vi "Aim_At_Target.vi"() -> ()   [LabVIEW 2019]
uses:
  <vilib>/Rock Robotics/WPI/Joystick/XBox Buttons Indexer.ctl
  <vilib>/Rock Robotics/WPI/Joystick/XBox Axes Indexer.ctl
  <vilib>/Rock Robotics/WPI/ThirdParty/JAS_Junk/TrajLib/PIDController_AtSetpoint.vi
  <vilib>/Rock Robotics/WPI/ThirdParty/JAS_Junk/TrajLib/PIDController_SetPIDF.vi
  <vilib>/Rock Robotics/WPI/ThirdParty/JAS_Junk/TrajLib/PIDController_SetDerivativeFilter.vi
  <vilib>/Rock Robotics/WPI/ThirdParty/JAS_Junk/TrajLib/PIDController_SetIntegratorRange.vi
  <vilib>/Rock Robotics/WPI/ThirdParty/JAS_Junk/TrajLib/PIDController_SetTolerancePandV.vi
  <vilib>/Rock Robotics/WPI/ThirdParty/JAS_Junk/TrajLib/PIDController_DisableContinousInput.vi
  <vilib>/Rock Robotics/WPI/ThirdParty/JAS_Junk/TrajLib/PIDController_EnableContinousInput.vi
  <vilib>/Rock Robotics/WPI/ThirdParty/JAS_Junk/TrajLib/PIDController_Reset.vi
  <vilib>/Rock Robotics/WPI/ThirdParty/JAS_Junk/TrajLib/PIDController_New.vi
  <vilib>/Rock Robotics/WPI/ThirdParty/JAS_Junk/TrajLib/PIDController_SetOutputLimits.vi
  <vilib>/Rock Robotics/WPI/ThirdParty/JAS_Junk/TrajLib/PIDController_NewPeriod.vi
  <vilib>/Rock Robotics/SystemInterfaces/NetworkCommunication/NetComm_UsageReport_report.vi
  <vilib>/Rock Robotics/WPI/Utilities/WPI_GetSetVariantRefNum.vi
  <vilib>/Rock Robotics/Network Tables/NT Write Boolean.vi
  <vilib>/Rock Robotics/WPI/Joystick/WPI_JoystickArcadeMapping.vi
  <vilib>/Rock Robotics/Network Tables/NT Write Number.vi
  <vilib>/Rock Robotics/WPI/ThirdParty/JAS_Junk/TrajLib/Util_LibraryGlobals.vi
  <vilib>/Rock Robotics/WPI/ThirdParty/JAS_Junk/TrajLib/PIDController_AdvCalculate_FF_Sp_Pv.vi
  <vilib>/Rock Robotics/Network Tables/NT Write Numeric Array.vi
  <vilib>/Rock Robotics/WPI/ThirdParty/PhotonVisionLib/PhotonVisionLib.lvlib
  <vilib>/Rock Robotics/WPI/ThirdParty/JAS_Junk/TrajLib/Trajectory_Library.lvlib
panel:
  in  "Fiiducial ID":i32
  in  "Use Fiducial\nID":bool
  out "Auto Aim\nSelected":bool
  out "TargetFound":bool
  out "Yaw":dbl
  out "DistanceToTarget Meters":dbl
  out "Right Motor Demand":dbl format="%14.4f"
  out "Left Motor Demand":dbl format="%14.4f"
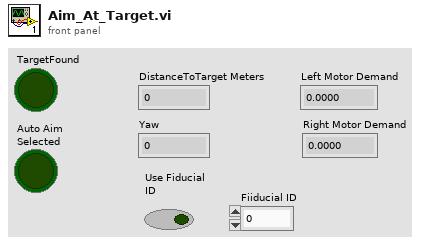
[diagram p1: front panel]
types:
  T1 = typedef "WPI_RobotDriveDevRef.ctl" = cluster{"DevStatus":errorcluster, "Motors[]":T2[], "Square Inputs":bool, "Max Output":dbl}
  T2 = typedef "WPI_MotorControlDeviceRef.ctl" = cluster{"DeviceStatus":errorcluster, "Type":T3, "PWM":cluster{"PWM Channel":T4, "DeadBand":T5}, "CAN":cluster{"Device Number":u8, "SetOutput VI Ref":variant, "GetOutput VI Ref":variant, "Enable VI Ref":variant, "Disable VI Ref":variant, "Data":variant}, "Invert":bool, "DIO PWM":cluster{"PWM \"Enable\" Channel":T4, "DIOChannel":T6, "PWM Rate":dbl}}
  T3 = typedef "WPI_MotorControlType.ctl" = enum16{"PWM", "CAN", "DIO PWM"}
  T4 = typedef "FPGA_DIOPWMChannel.ctl" = enum8{"PWM 0", "PWM 1", "PWM 2", "PWM 3", "PWM 4", "PWM 5", "PWM 6", "PWM 7", "PWM 8", "PWM 9", "PWM MXP 0", "PWM MXP 1", "PWM MXP 2", "PWM MXP 3", "PWM MXP 4", "PWM MXP 5", "PWM MXP 6", "PWM MXP 7", "PWM MXP 8", "PWM MXP 9", "Invalid"}
  T5 = typedef "WPI_PWMDeadband.ctl" = cluster{"Name":string, "maxPositivePwm":i32, "minPositivePwm":i32, "centerPwm":i32, "maxNegativePwm":i32, "minNegativePwm":i32, "angularRange":u16}
  T6 = typedef "FPGA_DIOChannel.ctl" = enum8{"DIO 0", "DIO 1", "DIO 2", "DIO 3", "DIO 4", "DIO 5", "DIO 6", "DIO 7", "DIO 8", "DIO 9", "DIO MXP 0", "DIO MXP 1", "DIO MXP 2", "DIO MXP 3", "DIO MXP 4", "DIO MXP 5", "DIO MXP 6", "DIO MXP 7", "DIO MXP 8", "DIO MXP 9", "DIO MXP 10", "DIO MXP 11", "DIO MXP 12", "DIO MXP 13", "DIO MXP 14", "DIO MXP 15", "SPI Port CS1", "SPI Port CS2", "SPI Port CS3", "SPI Port MISO", "SPI Port MOSI", "Invalid"}
  T7 = typedef "WPI_JoystickDevRef.ctl" = cluster{"Device":T8}
  T8 = typedef "WPI_JoystickDeviceEnum.ctl" = enum16{"USB 0", "USB 1", "USB 2", "USB 3", "USB 4", "USB 5"}
  T9 = typedef "XBox Axes Indexer.ctl" = enum16{"Left X", "Left Y", "Left Trigger", "Right Trigger", "Right X", "Right Y"}
  T10 = typedef "XBox Buttons Indexer.ctl" = enum16{"A", "B", "X", "Y", "Left Bumper", "Right Bumper", "Back", "Start", "Left Joystick", "Right Joystick"}
  T11 = typedef "PhotonVisionLib.lvlib/PhotonPipelineResultType.ctl" = cluster{"TargetCount":i32, "Latency_MilliSec":dbl, "Targets":T12[], "TimeStampSec":dbl}
  T12 = typedef "PhotonVisionLib.lvlib/PhotonTrackedTargetType.ctl" = cluster{"Yaw":dbl, "Pitch":dbl, "Area":dbl, "Skew":dbl, "MinAreaRectCorners":T13[], "BestCameraToTarget":T14, "FiiducialId":i32, "AltCameraToTarget":T14, "PoseAmbiguity":dbl, "DetectedCorners":T13[]}
  T13 = typedef "PhotonVisionLib.lvlib/TargetCornerType.ctl" = cluster{"X":dbl, "Y":dbl}
  T14 = typedef "Trajectory_Library.lvlib/TRANSFORM3D.ctl" = cluster{"TRANSLATION3D":T15, "ROTATION3D":T16, "XF":bool}
  T15 = typedef "Trajectory_Library.lvlib/TRANSLATION3D.ctl" = cluster{"X":dbl, "Y":dbl, "Z":dbl}
  T16 = typedef "Trajectory_Library.lvlib/ROTATION3D.ctl" = cluster{"Q_quaternion":T17}
  T17 = typedef "Trajectory_Library.lvlib/QUATERNION.ctl" = cluster{"R":dbl, "V":dbl[]}
  T18 = typedef "Trajectory_Library.lvlib/PID_ADV_LIMITS.ctl" = cluster{"MaxInput":dbl, "MinInput":dbl, "Continuous":bool, "MaxOutput":dbl, "MinOutput":dbl}
  T19 = typedef "Trajectory_Library.lvlib/PID_ADV_TUNING.ctl" = cluster{"Kf":dbl, "Kp":dbl, "Ki":dbl, "Kd":dbl, "MaximumIntegral":dbl, "MinimumIntegral":dbl, "Filter Derivative":bool}
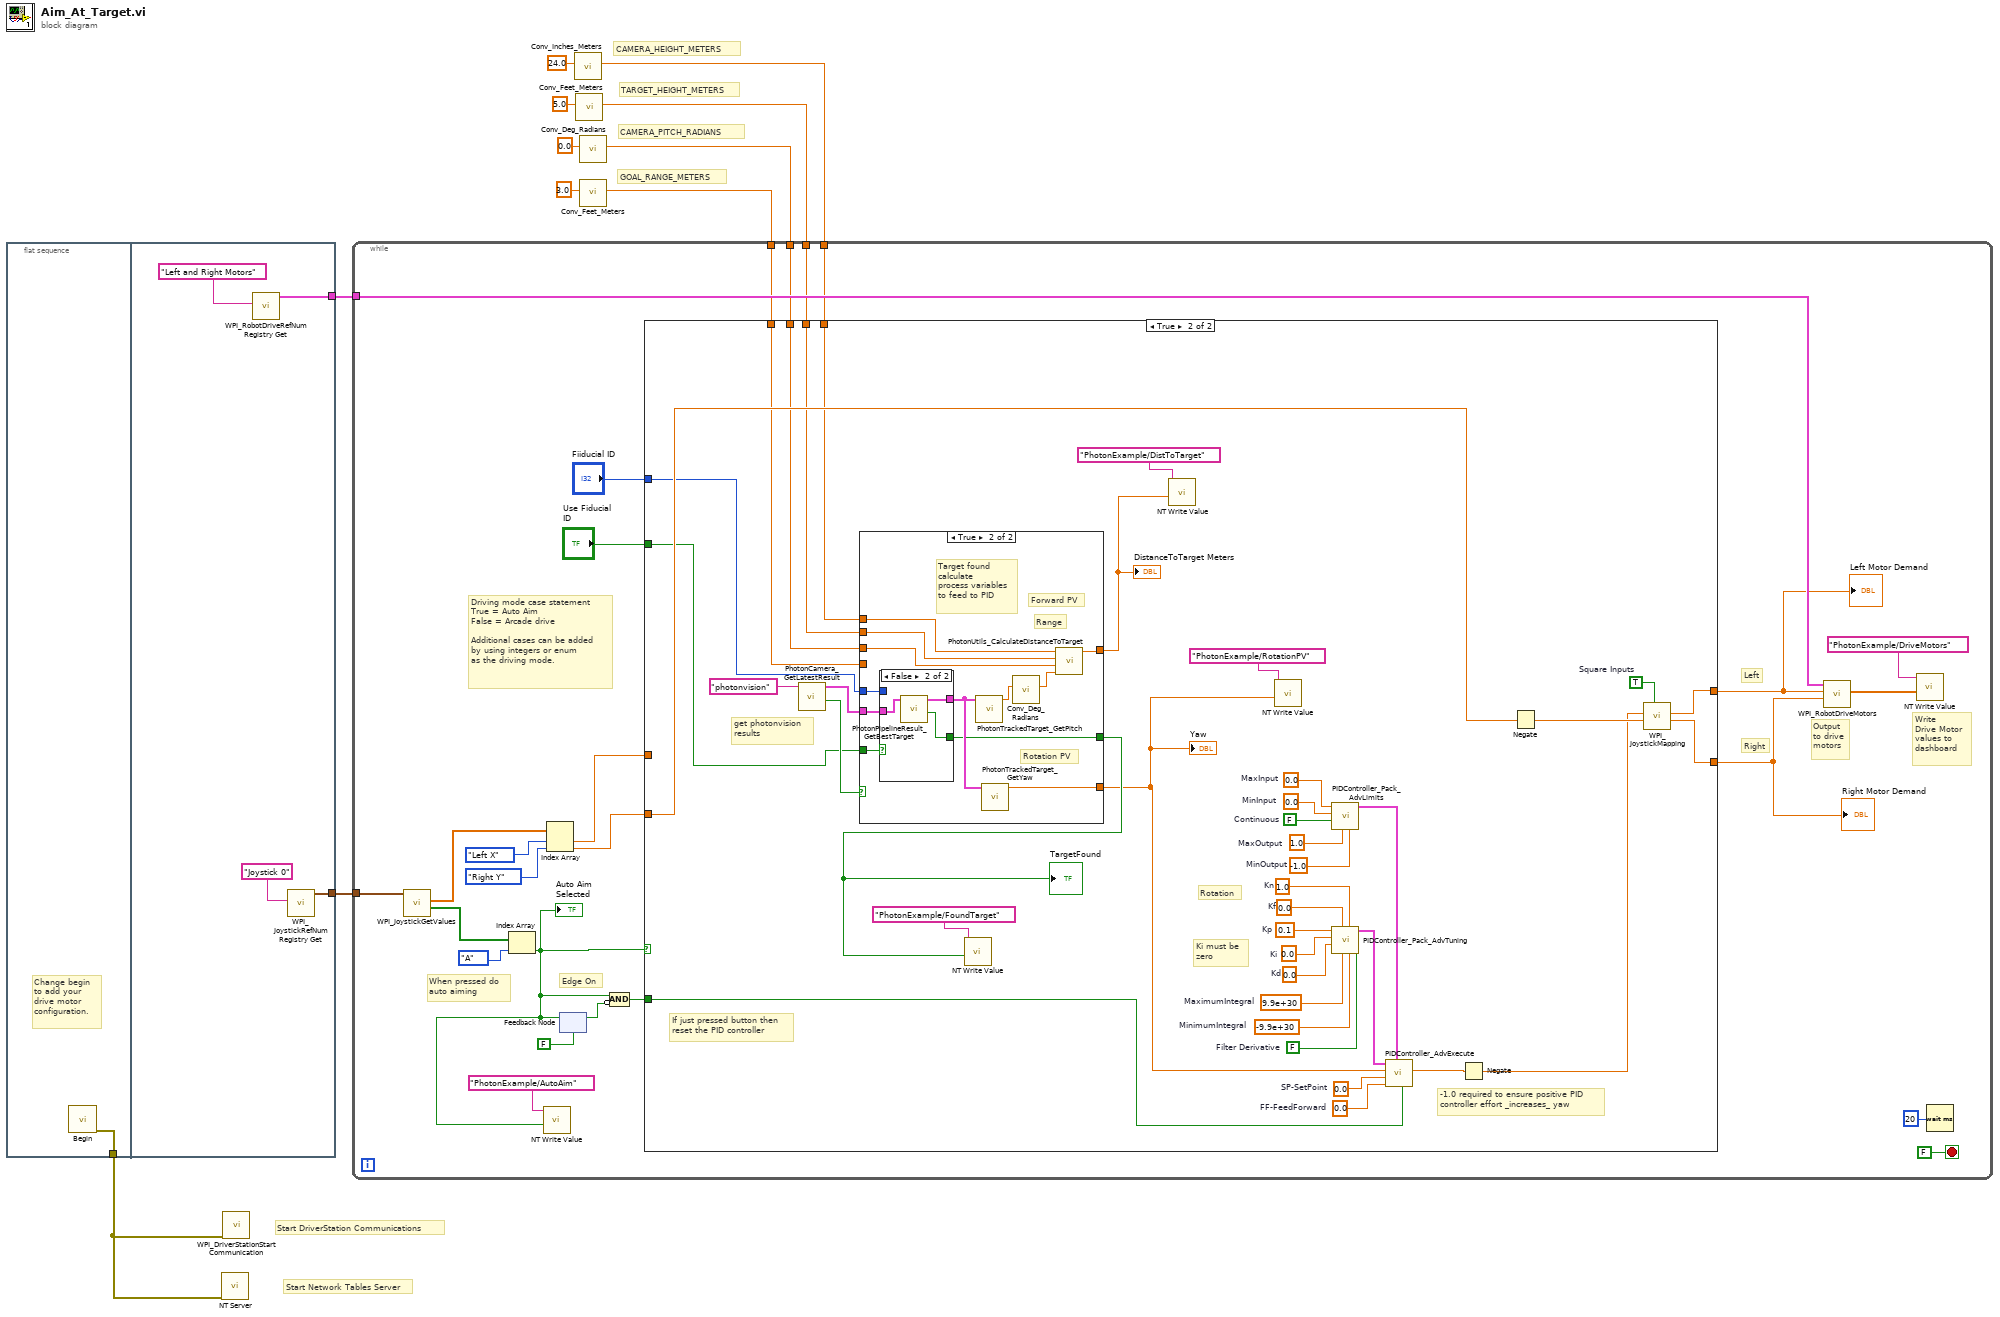
[diagram p0: block diagram]
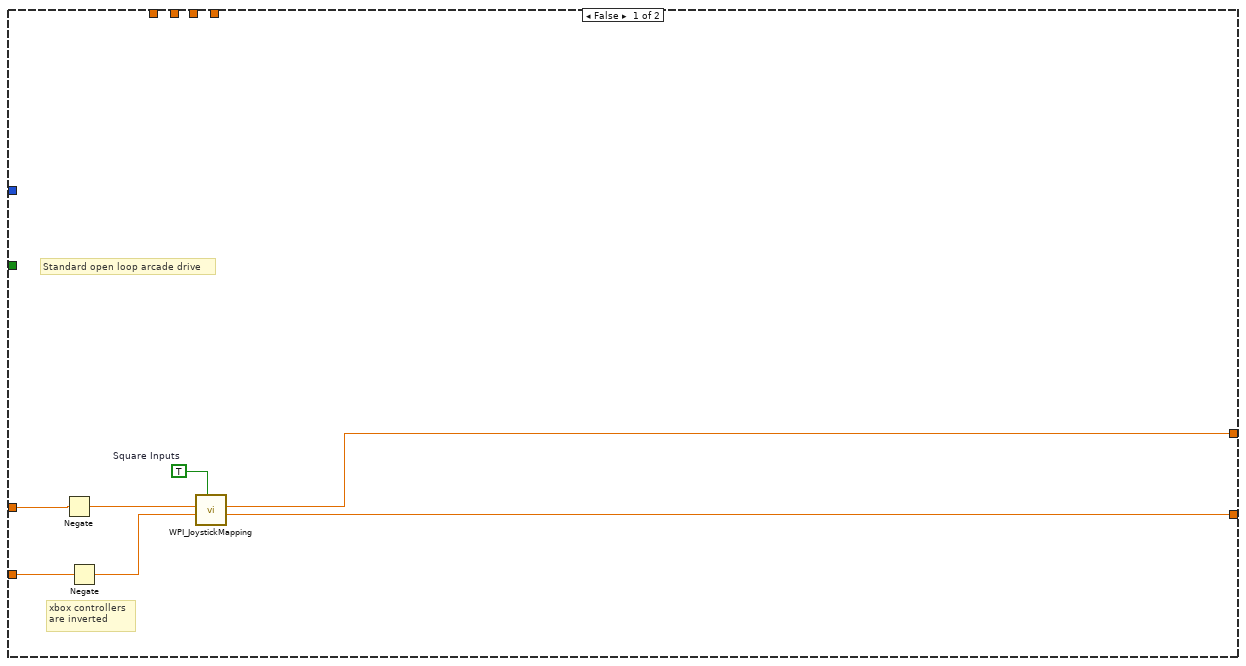
[diagram p2: hidden frame]
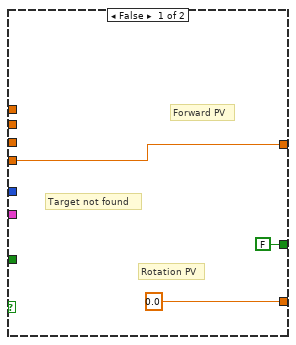
[diagram p3: hidden frame]
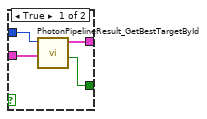
[diagram p4: hidden frame]
diagram:
  # "GOAL_RANGE_METERS"
  # "CAMERA_PITCH_RADIANS"
  # "TARGET_HEIGHT_METERS"
  # "CAMERA_HEIGHT_METERS"
  # "Start Network Tables Server"
  # "Start DriverStation Communications"
  n1 = flat-sequence {
    tunnel: [w12] -> w11
    tunnel: [w15] -> w10
    tunnel: [w13] -> w9
    frame #0 {
      # "Change begin\nto add your \ndrive motor\nconfiguration."
      n2 = call "Begin.vi"() -> ("error out"=w12:errorcluster)  [unwired: 11 in]
    }
    frame #1 {
      n3 = call <vilib>:"WPI_RobotDriveRefNum Registry Get.vi"("refnum name"="Left and Right Motors") -> ("RobotDriveDevRef"=w13:T1)  [unwired: 9 in, 1 out]
      n4 = call <vilib>:"WPI_JoystickRefNum Registry Get.vi"("refnum name"="Joystick 0") -> ("JoystickDevRef"=w15:T7)  [unwired: 9 in, 1 out]
    }
  }
  n5 = call <vilib>:"NT Server.vi"("error in (no error)"=w11) -> ()  [unwired: 11 in]
  n6 = call <vilib>:"WPI_DriverStationStart Communication.vi"("error in (no error)"=w11) -> ()  [unwired: 11 in]
  n7 = call <vilib>:"Conv_Inches_Meters.vi"("INCH"=24.0) -> ("Meters"=w4:dbl)  [unwired: 10 in]
  n8 = call <vilib>:"Conv_Feet_Meters.vi"("Feet"=5.0) -> ("Meters"=w3:dbl)  [unwired: 10 in]
  n9 = call <vilib>:"Conv_Feet_Meters.vi"("Feet"=3.0) -> ("Meters"=w1:dbl)  [unwired: 10 in]
  n10 = call <vilib>:"Conv_Deg_Radians.vi"("Degress"=0.0) -> ("Radians"=w2:dbl)  [unwired: 10 in]
  n11 = while {
    tunnel: w10 -> [w41]
    tunnel: w9 -> [w33]
    tunnel: w4 -> [w24]
    tunnel: w3 -> [w23]
    tunnel: w2 -> [w22]
    tunnel: w1 -> [w21]
    stop <- FALSE stop-if-true
    # "Write \nDrive Motor\nvalues to \ndashboard"
    # "Output\nto drive\nmotors"
    # "Edge On"
    # "Right"
    # "Left"
    # "Driving mode case statement\nTrue = Auto Aim\nFalse = Arcade drive\n\nAdditional cases can be added\nby using integers or enum\nas the driving mode."
    # "When pressed do\nauto aiming"
    n12 = call <vilib>:"WPI_JoystickGetValues.vi"("JoystickDevRef"=w41) -> ("Buttons"=w40:bool[], "Axes"=w39:dbl[])  [unwired: 6 in, 3 out]
    n13 = Index Array(array=w40, index=XBox_Buttons_Indexer."A" ("XBox Buttons")) -> (element=w19:bool)
    "Auto Aim\nSelected" <- w19
    n14 = call-poly <vilib>:"NT Write Value.vi"("Boolean"=w19, "Name"="PhotonExample/AutoAim") -> ()  [unwired: 9 in, 1 out]
    n15 = Index Array(array=w39, index #1=XBox_Axes_Indexer."Left X" ("XBox Axes"), index #2=XBox_Axes_Indexer."Right Y" ("XBox Axes")) -> (element #1=w35:dbl, element #2=w34:dbl)
    n16 = feedback-in #1(w19) -> ()
    n17 = feedback #1(FALSE) -> (w30:bool)
    n18 = Compound Arithmetic op=AND(w19, invert w30) -> (w31:bool)
    n19 = case shown="True" w19 {
      tunnel: w35 -> [w49 _]
      tunnel: w34 -> [w48 w61]
      tunnel: [w44 w87] -> w32
      tunnel: [w43 w86] -> w25
      tunnel: w31 -> [_ w69]
      tunnel: w24 -> [_ w56]
      tunnel: w23 -> [_ w55]
      tunnel: w22 -> [_ w54]
      tunnel: w21 -> [_ w53]
      tunnel: "Fiiducial ID" -> [_ w59]
      tunnel: "Use Fiducial\nID" -> [_ w50]
      frame False {
        w45 = TRUE  # Square Inputs
        # "Standard open loop arcade drive"
        # "xbox controllers\nare inverted"
        n20 = Negate(x=w49) -> (-x=w47:dbl)
        n21 = Negate(x=w48) -> (-x=w46:dbl)
        n22 = call-poly <vilib>:"WPI_JoystickMapping.vi"("Square Inputs"=w45, "Y axis value"=w46, "X axis value"=w47) -> ("Right Motor Value"=w43:dbl, "Left Motor Value"=w44:dbl)  [unwired: 7 in]
      }
      frame True {
        w68 = 0.0  # FF-FeedForward
        w70 = 0.0  # SP-SetPoint
        w85 = 1.0  # Kn
        w84 = 0.1  # Kp
        w83 = 0.0  # Ki
        w82 = 0.0  # Kd
        w81 = 0.0  # Kf
        w80 = 9.9e+30  # MaximumIntegral
        w79 = -9.9e+30  # MinimumIntegral
        w78 = FALSE  # Filter Derivative
        w76 = 0.0  # MinInput
        w75 = FALSE  # Continuous
        w74 = 1.0  # MaxOutput
        w77 = -1.0  # MinOutput
        w73 = 0.0  # MaxInput
        w88 = TRUE  # Square Inputs
        # "-1.0 required to ensure positive PID \ncontroller effort _increases_ yaw"
        # "Ki must be \nzero"
        # "If just pressed button then\nreset the PID controller"
        # "Rotation"
        # "get photonvision\nresults"
        n23 = call <vilib>:"PhotonCamera_GetLatestResult.vi"("CameraName"="photonvision") -> ("HasTargets"=w58:bool, "PipelineResult"=w60:T11)  [unwired: 9 in]
        n24 = case shown="True" w58 {
          tunnel: w60 -> [_ w104]
          tunnel: [w91 w100] -> w52
          tunnel: [0.0 w99] -> w51
          tunnel: w56 -> [_ w96]
          tunnel: w55 -> [_ w97]
          tunnel: w54 -> [_ w98]
          tunnel: w53 -> [w91 _]
          tunnel: w50 -> [_ w95]
          tunnel: [FALSE ("TargetFound") w94] -> w57
          tunnel: w59 -> [_ w93]
          frame False {
            # "Forward PV"
            # "Rotation PV"
            # "Target not found"
          }
          frame True {
            # "Target found\ncalculate\nprocess variables\nto feed to PID"
            # "Range"
            # "Forward PV"
            # "Rotation PV"
            n25 = case shown="False" w95 {
              tunnel: w104 -> [w106 w111]
              tunnel: [w108 w110] -> w101
              tunnel: [w107 w109] -> w94
              tunnel: w93 -> [w105 _]
              frame True {
                n26 = call <vilib>:"PhotonPipelineResult_GetBestTargetById.vi"("PhotonPipelineResult"=w106, "FiducialId"=w105) -> ("Target Found"=w107:bool, "PhotonTrackedTarget"=w108:T12)  [unwired: 7 in, 1 out]
              }
              frame False {
                n27 = call <vilib>:"PhotonPipelineResult_GetBestTarget.vi"("PhotonPipelineResult"=w111) -> ("TargetFound"=w109:bool, "PhotonTrackedTarget"=w110:T12)  [unwired: 9 in]
              }
            }
            n28 = call <vilib>:"PhotonTrackedTarget_GetPitch.vi"("TrackedTarget"=w101) -> ("Pitch"=w103:dbl)  [unwired: 10 in]
            n29 = call <vilib>:"PhotonTrackedTarget_GetYaw.vi"("TrackedTarget"=w101) -> ("Yaw"=w99:dbl)  [unwired: 10 in]
            n30 = call <vilib>:"Conv_Deg_Radians.vi"("Degress"=w103) -> ("Radians"=w102:dbl)  [unwired: 10 in]
            n31 = call <vilib>:"PhotonUtils_CalculateDistanceToTarget.vi"("TargetPitch_Radians"=w102, "CameraPitch_Radians"=w98, "TargetHeight_Meters"=w97, "CameraHeight_Meters"=w96) -> ("DistanceToTarget_Meters"=w100:dbl)  [unwired: 7 in]
          }
        }
        "DistanceToTarget Meters" <- w52
        "Yaw" <- w51
        "TargetFound" <- w57
        n32 = call-poly <vilib>:"NT Write Value.vi"("Boolean"=w57, "Name"="PhotonExample/FoundTarget") -> ()  [unwired: 9 in, 1 out]
        n33 = call-poly <vilib>:"NT Write Value.vi"("Numeric"=w52, "Name"="PhotonExample/DistToTarget") -> ()  [unwired: 9 in, 1 out]
        n34 = call-poly <vilib>:"NT Write Value.vi"("Numeric"=w51, "Name"="PhotonExample/RotationPV") -> ()  [unwired: 9 in, 1 out]
        n35 = call <vilib>:"PIDController_Pack_AdvLimits.vi"("MinOutput"=w77, "MaxOutput"=w74, "Continuous"=w75, "MinInput"=w76, "MaxInput"=w73) -> ("Adv PID Limits"=w71:T18)  [unwired: 6 in]
        n36 = call <vilib>:"PIDController_Pack_AdvTuning.vi"("Filter Derivative"=w78, "MinimumIntegral"=w79, "Kn"=w85, "MaximumIntegral"=w80, "Kf"=w81, "Kd"=w82, "Ki"=w83, "Kp"=w84) -> ("Adv PID Tuning"=w72:T19)  [unwired: 3 in]
        n37 = call <vilib>:"PIDController_AdvExecute.vi"("Reset"=w69, "Adv PID Limits"=w71, "FF-FeedForward"=w68, "SP-SetPoint"=w70, "PV-Measurement"=w51, "Adv PID Tuning"=w72) -> ("CO-ControlOutput"=w66:dbl)  [unwired: 3 in, 2 out]
        n38 = Negate(x=w66) -> (-x=w65:dbl)
        n39 = Negate(x=w61) -> (-x=w67:dbl)
        n40 = call-poly <vilib>:"WPI_JoystickMapping.vi"("Square Inputs"=w88, "Y axis value"=w67, "X axis value"=w65) -> ("Right Motor Value"=w86:dbl, "Left Motor Value"=w87:dbl)  [unwired: 7 in]
      }
    }
    "Left Motor Demand" <- w32
    "Right Motor Demand" <- w25
    n41 = call <vilib>:"WPI_RobotDriveMotors.vi"("RightSpeed"=w25, "LeftSpeed"=w32, "RobotDriveDevRef"=w33) -> ("Motor Values"=w27:dbl[])  [unwired: 6 in, 2 out]
    n42 = call-poly <vilib>:"NT Write Value.vi"("Numeric Array"=w27, "Name"="PhotonExample/DriveMotors") -> ()  [unwired: 9 in, 1 out]
    n43 = Wait (ms)(milliseconds to wait=u32 20) -> ()  [unwired: 1 out]
  }
